vi "Write flows.vi"(8 "error in (no error)":errorcluster, 10 "flows":bool, 11 "Set Flows for Blue in":refnum<class "Set Flows for Blue.lvclass">) -> (0 "error out":errorcluster, 3 "Set Flows for Blue out":refnum<class "Set Flows for Blue.lvclass">)   [LabVIEW 2013, in "Set Flows for Blue.lvclass"]
uses:
  Set Flows for Blue.lvclass
  Set Flows for Blue.lvclass/Set Flows for Blue.ctl
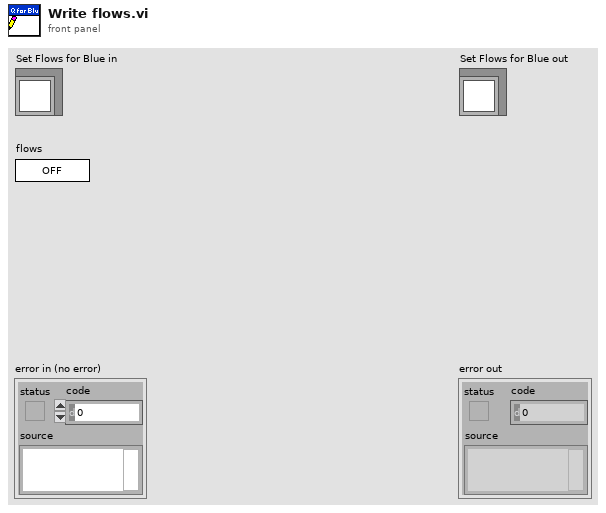
[diagram p1: front panel]
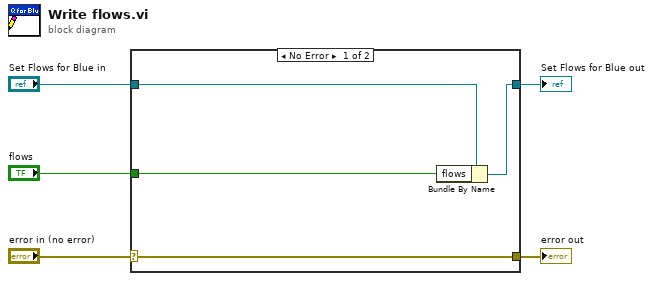
[diagram p0: block diagram]
diagram:
  n1 = case shown="No Error" "error in (no error)" {
    selector: "error in (no error)" -> [w9 w10]
    tunnel: [w9 w10] -> w4
    tunnel: [w7 w11] -> w2
    tunnel: "Set Flows for Blue in" -> [w8 w11]
    tunnel: "flows" -> [w6 _]
    frame No Error {
      n2 = Bundle By Name(cluster=w8, "flows"=w6) -> (w7:refnum<class "Set Flows for Blue.lvclass">)
    }
    frame Error {
    }
  }
  "error out" <- w4
  "Set Flows for Blue out" <- w2
